vi "Main.vi"(5 "Deliminated Char":string=".", 6 "Folder names":string[](array[string])=["StaARx#[PLC]StaATesterRxSignals", "StaATx#[PLC]StaATesterTxSignals"], 7 "PLC FGVname":string="OPC Ref", 8 "error in":errorcluster, 9 "Sequence Context In":refnum<k7>, 10 "Event Sources":T1, 11 "TestExec In":refnum<class "TestExec.lvclass">) -> (0 "error out":errorcluster, 2 "Station":string, 3 "TestExec Out":refnum<class "TestExec.lvclass">)   [LabVIEW 2021, in "TestExec.lvclass"]
uses:
  TestExec.lvclass
  Controls/Rx TestExec.ctl
  Controls/Tx TestExec.ctl
  TestExec.lvclass/TestExec.ctl
  Methods/Cylinder Display.vi
  <vilib>/addons/TestStand/_TSUtility.llb/TestStand - Get Property Value (Number {Signed 32-bit Integer}).vi
  OPC UA/OPC UA.lvclass
panel:
  out "Connect":bool
  in  "Tx TestExec":T2={"HighVoltage"=TRUE, "TestRunning"=FALSE, "StepNo"=0, "Fault"=FALSE}
  out "Rx TestExec":T3
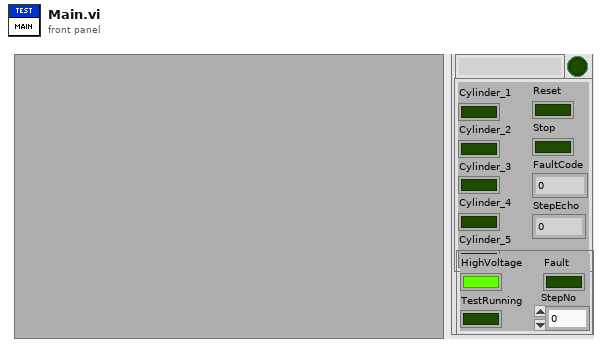
[diagram p1: front panel]
types:
  T1 = cluster{"Stop":refnum<user-event>, "Variant":refnum<user-event>}
  T2 = typedef "TestExec.lvclass/Tx TestExec.ctl" = cluster{"HighVoltage":bool, "TestRunning":bool, "StepNo":u32, "Fault":bool}
  T3 = typedef "TestExec.lvclass/Rx TestExec.ctl" = cluster{"Cylinder_1":bool, "Cylinder_2":bool, "Cylinder_3":bool, "Cylinder_4":bool, "Cylinder_5":bool, "StepEcho":u32, "Reset":bool, "Stop":bool, "FaultCode":u32}
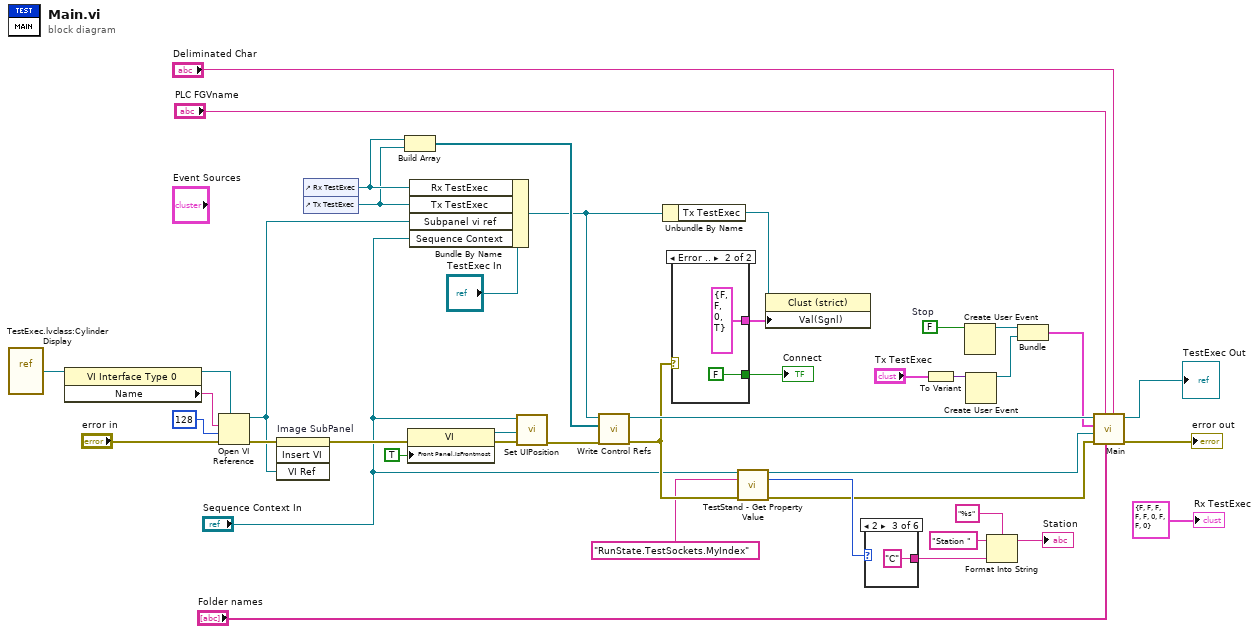
[diagram p0: block diagram]
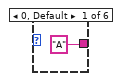
[diagram p2: hidden frame]
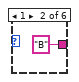
[diagram p3: hidden frame]
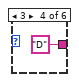
[diagram p4: hidden frame]
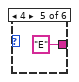
[diagram p5: hidden frame]
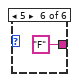
[diagram p6: hidden frame]
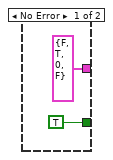
[diagram p7: hidden frame]
diagram:
  w31 = FALSE  # Stop
  n1 = vi-ref "TestExec.lvclass:Cylinder Display.vi"() -> (w24:refnum<vi>)
  n2 = property on="Property Node" class="VI Interface Type 0"(reference=w24) -> (reference out=w26:refnum<vi>, "Name"=w25:string)  [unwired: 1 in, 1 out]
  n3 = Open VI Reference(type specifier VI Refnum (for type only)=w26, vi path=w25, options=128, error in (no error)="error in") -> (vi reference=w19:refnum<vi>, error out=w21:errorcluster)  [unwired: 2 in]
  n4 = invoke on="Image SubPanel" class="SubPnl" method="Insert VI"(error in=w21, "VI Ref"=w19) -> (error out=w18:errorcluster)  [unwired: 2 in, 3 out]
  n5 = control-ref of="Rx TestExec"() -> (w36:refnum<vi>)
  n6 = control-ref of="Tx TestExec"() -> (w35:refnum<vi>)
  n7 = Build Array(w36, w35) -> (w34:refnum<vi>[])
  n8 = property class="VI"(error in=w18, "Front Panel.IsFrontmost"=TRUE ("Front Panel Window:Is Frontmost")) -> (reference out=w16:refnum<vi>, error out=w17:errorcluster)  [unwired: 1 in]
  n9 = Bundle By Name(cluster="TestExec In", "Rx TestExec"=w36, "Tx TestExec"=w35, "Subpanel vi ref"=w19, "Sequence Context"="Sequence Context In") -> (w33:refnum<class "TestExec.lvclass">)
  n10 = call "Set UIPosition.vi"("error in"=w17, "VI Ref"=w16, "Sequence Context In"="Sequence Context In") -> ("error out"=w15:errorcluster)  [unwired: 8 in]
  n11 = call-dynamic "Write Control Refs.vi"("error in (no error)"=w15, "Ctl Refs"=w34, "OPC UA in"=w33) -> ("error out"=w5:errorcluster, "OPC UA out"=w28:refnum<class "TestExec.lvclass">)  [unwired: 7 in]
  n12 = Unbundle By Name(w33) -> ("Tx TestExec"=w39:refnum<vi>)
  n13 = case shown="Error .." w5 {
    tunnel: [T2 {"HighVoltage"=FALSE, "TestRunning"=TRUE, "StepNo"=0, "Fault"=FALSE} ("Test Exec Tx") T2 {"HighVoltage"=FALSE, "TestRunning"=FALSE, "StepNo"=0, "Fault"=TRUE} ("Test Exec Tx")] -> w40
    tunnel: [TRUE ("Connect") FALSE ("Connect")] -> w37
    frame No Error {
    }
    frame Error {
    }
  }
  "Connect" <- w37
  n14 = call-poly <vilib>:"TestStand - Get Property Value.vi"("Sequence Context In"="Sequence Context In", "Lookup String"="RunState.TestSockets.MyIndex", "error in (no error)"=w5) -> ("Sequence Context Out"=w3:refnum<k7>, "Value"=w9:i32, "error out"=w4:errorcluster)  [unwired: 10 in]
  n15 = property class="Clust (strict)"(reference=w39, "Val(Sgnl)"=w40) -> ()  [unwired: 1 in, 2 out]
  n16 = case shown="2" w9 {
    tunnel: ["A" ("format string") "B" ("format string") "C" ("format string") "D" ("format string") "E" ("format string") "F" ("format string")] -> w10
    frame 0, Default {
    }
    frame 1 {
    }
    frame 2 {
    }
    frame 3 {
    }
    frame 4 {
    }
    frame 5 {
    }
  }
  n17 = To Variant(anything="Tx TestExec") -> (Variant=w42:variant)
  n18 = Create User Event(user event datatype=w31) -> (user event=w32:refnum<user-event>)  [unwired: 1 in, 1 out]
  n19 = Create User Event(user event datatype=w42) -> (user event=w30:refnum<user-event>)  [unwired: 1 in, 1 out]
  n20 = Format Into String(format string="%s", initial string="Station ", w10) -> (resulting string=→"Station":string)  [unwired: 1 in, 1 out]
  n21 = Bundle("Stop"=w32, "Variant"=w30) -> (w13:T1)  [unwired: 1 in]
  n22 = call-parent "Main.vi"("Deliminated Char"="Deliminated Char", "Folder names"="Folder names", "FGVname"="PLC FGVname", "error in"=w4, "Sequence Context In"=w3, "Event Sources"=w13, "OPC UA In"=w28) -> ("error out"=→"error out":errorcluster, "OPC UA Out"=→"TestExec Out":refnum<class "TestExec.lvclass">)  [unwired: 2 in, 1 out]
  "Rx TestExec" <- T3 {"Cylinder_1"=FALSE, "Cylinder_2"=FALSE, "Cylinder_3"=FALSE, "Cylinder_4"=FALSE, "Cylinder_5"=FALSE, "StepEcho"=0, "Reset"=FALSE, "Stop"=FALSE, "FaultCode"=0} ("Rx TestExec")
